vi "Create Memory Monitor Frame from Standard Out.vi"(11 "Starndard Output":string) -> (3 "Frame":variant)   [LabVIEW 2021]
uses:
  Type Definitions/Payload Class.ctl
  Type Definitions/Enumerated Constants/Software Monitor.ctl
  Type Definitions/Memory Monitor.ctl
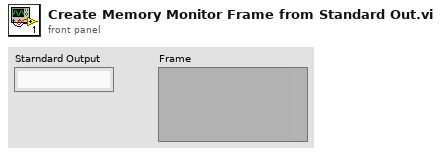
[diagram p1: front panel]
types:
  T1 = typedef "Memory Monitor.ctl" = cluster{"Total Memory":sgl, "Available Memory":sgl}
  T2 = typedef "Software Monitor.ctl" = enum16{"Internet Connection Monitor", "CPU Monitor", "Archive Monitor", "Memory Monitor", "Queue Monitor", "RTOS Update", "RTOS Monitor"}
  T3 = typedef "Payload Class.ctl" = enum16{"System State", "Parameters", "Metadata", "Software Monitor", "Data", "Commands"}
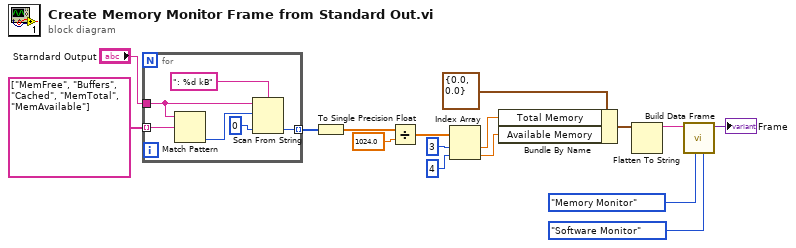
[diagram p0: block diagram]
diagram:
  n1 = for {
    tunnel: "Starndard Output" -> [w17]
    tunnel: string[] ["MemFree", "Buffers", "Cached", "MemTotal", "MemAvailable"] ("command line") -> [w22] mode=indexing
    tunnel: [w20] -> w6 mode=indexing
    n2 = Match Pattern(string=w17, regular expression=w22) -> (offset past match=w19:i32)  [unwired: 1 in, 3 out]
    n3 = Scan From String(format string=": %d kB", input string=w17, initial scan location=w19, default 1=u32 0) -> (output 1=w20:u32)  [unwired: 1 in, 3 out]
  }
  n4 = To Single Precision Float(number=w6) -> (single precision float=w8:sgl[])
  n5 = Divide(x=w8, y=sgl 1024.0) -> (x/y=w10:sgl[])
  n6 = Index Array(array=w10, index #1=3 ("index"), index #2=4 ("index")) -> (element #1=w14:sgl, element #2=w15:sgl)
  n7 = Bundle By Name(cluster=T1 {"Total Memory"=0.0, "Available Memory"=0.0}, "Total Memory"=w14, "Available Memory"=w15) -> (w4:T1)
  n8 = Flatten To String(anything=w4) -> (data string=w3:string)  [unwired: 3 in, 2 out]
  n9 = call "Build Data Frame.vi"("Payload Class (Data)"=Payload_Class."Software Monitor", "Payload ID (0)"=Software_Monitor."Memory Monitor", "Payload (Empty String)"=w3) -> ("Frame"=→"Frame":variant)  [unwired: 7 in, 1 out]
